vi "Not a Num Primitive String.vi"() -> (3 "Error":string)   [LabVIEW 2017]
uses:
  _Shared/CSM Shared.lvlib
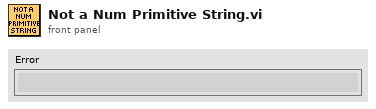
[diagram p1: front panel]
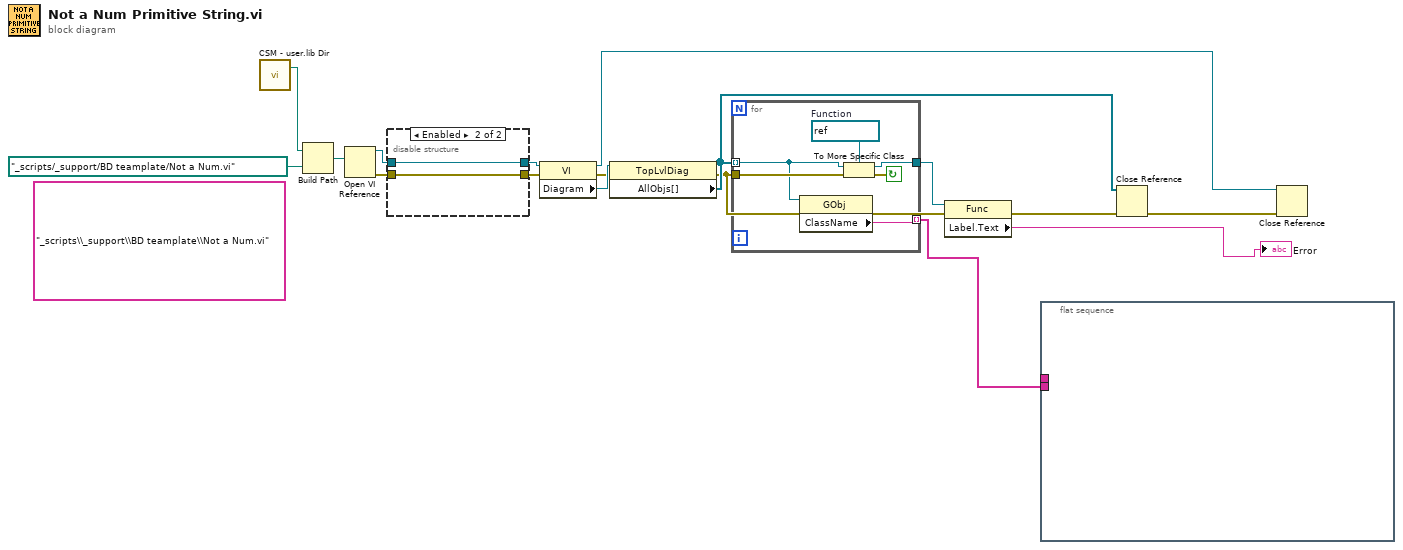
[diagram p0: block diagram]
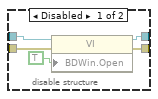
[diagram p2: hidden frame]
diagram:
  (unwired) "_scripts\\_support\\BD teamplate\\Not a Num.vi" ("name or relative path")
  n1 = call "CSM - user.lib Dir.vi"() -> ("csm_user.lib_dir"=w8:path)  [unwired: 2 in, 1 out]
  n2 = Build Path ("创建路径")(base path=w8, name or relative path=path "_scripts/_support/BD teamplate/Not a Num.vi") -> (appended path=w9:path)
  n3 = Open VI Reference ("打开VI引用")(vi path=w9) -> (vi reference=w7:refnum<vi>, error out=w6:errorcluster)  [unwired: 5 in]
  n4 = disable-structure "程序框图禁用结构" shown="Enabled" {
    disable-tunnel: w7 -> [w22 w24]
    disable-tunnel: w6 -> [w21 w23]
    disable-tunnel: [w20 w24] -> w17
    disable-tunnel: [w19 w23] -> w16
    frame Disabled {
      n5 = property class="VI"(reference=w22, error in=w21, "BDWin.Open"=TRUE ("Block Diagram Window:Open")) -> (reference out=w20:refnum<vi>, error out=w19:errorcluster)
    }
    frame Enabled {
    }
  }
  n6 = property on="属性节点" class="VI"(reference=w17, error in=w16) -> (reference out=w12:refnum<vi>, error out=w14:errorcluster, "Diagram"=w15:refnum<vi>)
  n7 = property on="属性节点" class="TopLvlDiag"(reference=w15, error in=w14) -> (error out=w10:errorcluster, "AllObjs[]"=w11:refnum<vi>[])  [unwired: 1 out]
  n8 = for "For循环" {
    tunnel: w11 -> [w26] mode=indexing
    tunnel: [w27] -> w13
    tunnel: w10 -> [w29]
    tunnel: [w25] -> w3 mode=indexing
    stop <- w28 continue-if-true
    w30 = refnum<vi> refnum  # Function
    n9 = property on="属性节点" class="GObj"(reference=w26) -> ("ClassName"=w25:string)  [unwired: 1 in, 2 out]
    n10 = To More Specific Class(target class=w30, reference=w26, error in=w29) -> (specific class reference=w27:refnum<vi>, error out=w28:errorcluster)
  }
  n11 = property on="属性节点" class="Func"(reference=w13, error in=w10) -> (error out=w5:errorcluster, "Label.Text"=→"Error":string)  [unwired: 1 out]
  n12 = flat-sequence {
    tunnel: [w31] -> _
    tunnel: w3 -> [w31]
    frame #0 {
    }
  }
  n13 = Close Reference ("关闭引用")(reference=w11, error in (no error)=w5) -> (error out=w4:errorcluster)
  n14 = Close Reference ("关闭引用")(reference=w12, error in (no error)=w4) -> ()  [unwired: 1 out]
